vi "Update Label.vi"(8 "error in":errorcluster, 10 "label value":u8 format="%.0o", 11 "32-bit word in":refnum<class "32-bit Word.lvclass">) -> (0 "error out":errorcluster, 3 "32-bit word out":refnum<class "32-bit Word.lvclass">)   [LabVIEW 2020, in "32-bit Word.lvclass"]
uses:
  32-bit Word.lvclass
  C:/Git/niveristand-communications-bus-template/Source/Protocol/Implementations/ARINC429/ARINC 429.lvclass
  32-bit Word.lvclass/32-bit Word.ctl
  ARINC 429.lvclass/ARINC 429.ctl
  5c5fc4fb-6106-4363-aed5-f97f5350a028.vi
  Read 32-Bit Word.vi
  Read Label Start Index.vi
  Read Label Size.vi
  Write 32-Bit Word.vi
  Write Label Value.vi
  5c5fc4fb-6106-4363-aed5-f97f5350a028.vi/a7fcce85-1f75-4572-aeaa-ddfd463a7c5f.vi
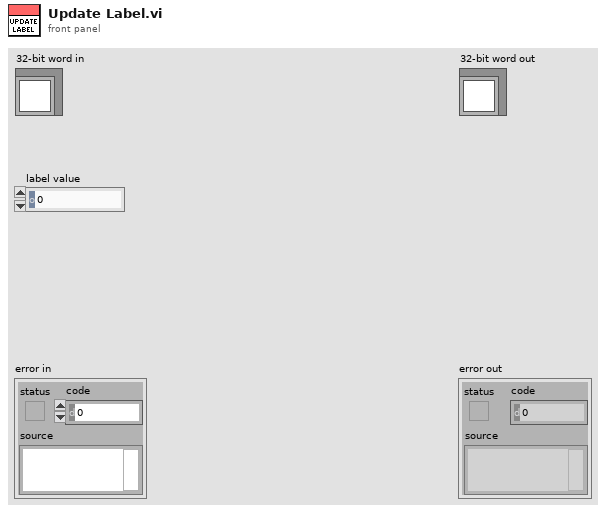
[diagram p1: front panel]
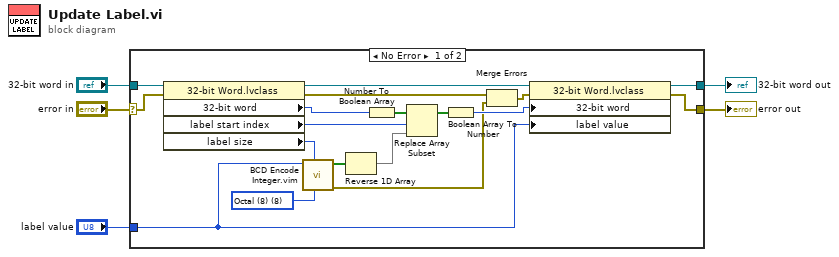
[diagram p0: block diagram]
diagram:
  n1 = case shown="No Error" "error in" {
    selector: "error in" -> [w10 w25]
    tunnel: [w9 w25] -> w4
    tunnel: [w14 w24] -> w2
    tunnel: "32-bit word in" -> [w13 w24]
    tunnel: "label value" -> [w6 _]
    frame No Error {
      w22 = u8 8 items=["Binary (2)"=2, "Octal (8)"=8, "Decimal (10)"=10, "Hexadecimal (16)"=16] ("base")
      n2 = property on="Property Node" class="32-bit Word.lvclass"(reference=w13, error in=w10) -> (reference out=w15:refnum<class "32-bit Word.lvclass">, error out=w11:errorcluster, "32-bit word"=w21:u32, "label start index"=w18:i32, "label size"=w23:i32)
      n3 = call "BCD Encode Integer.vim"("base"=w22, "data size (bits)"=w23, "integer"=w6) -> ("error out"=w7:errorcluster, "BCD encoded value"=w19:bool[])  [unwired: 7 in]
      n4 = Reverse 1D Array(array=w19) -> (reversed array=w12:bool[])
      n5 = Number To Boolean Array(number=w21) -> (Boolean array=w20:bool[])
      n6 = Replace Array Subset(array=w20, new element=w12, index=w18) -> (w17:bool[])
      n7 = Boolean Array To Number(Boolean array=w17) -> (number=w16:u32)
      n8 = Merge Errors(w11, w7) -> (w8:errorcluster)
      n9 = property on="Property Node" class="32-bit Word.lvclass"(reference=w15, error in=w8, "32-bit word"=w16, "label value"=w6) -> (reference out=w14:refnum<class "32-bit Word.lvclass">, error out=w9:errorcluster)
    }
    frame Error {
    }
  }
  "error out" <- w4
  "32-bit word out" <- w2
